vi "GetParameterValueInteger.vi"(8 "error in (no error)":errorcluster, 11 "Parameter in":refnum<class "Parameter.lvclass">) -> (0 "error out":errorcluster, 2 "Value":i32, 3 "Parameter out":refnum<class "Parameter.lvclass">)   [LabVIEW 2023, in "Easy.SequenceManagerLabVIEW.lvlib" / "Parameter.lvclass"]
uses:
  Parameter.lvclass
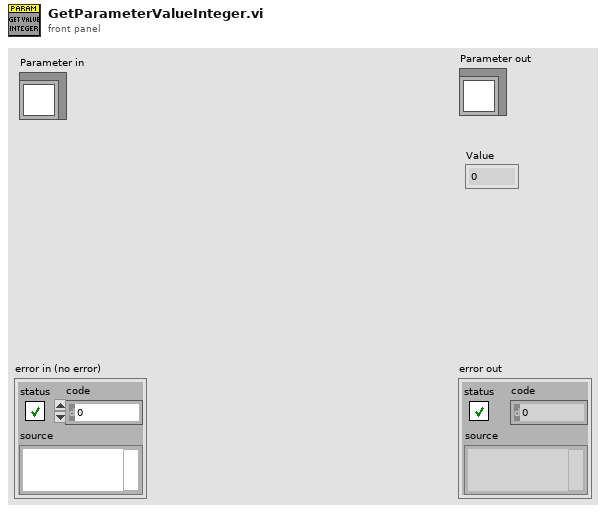
[diagram p1: front panel]
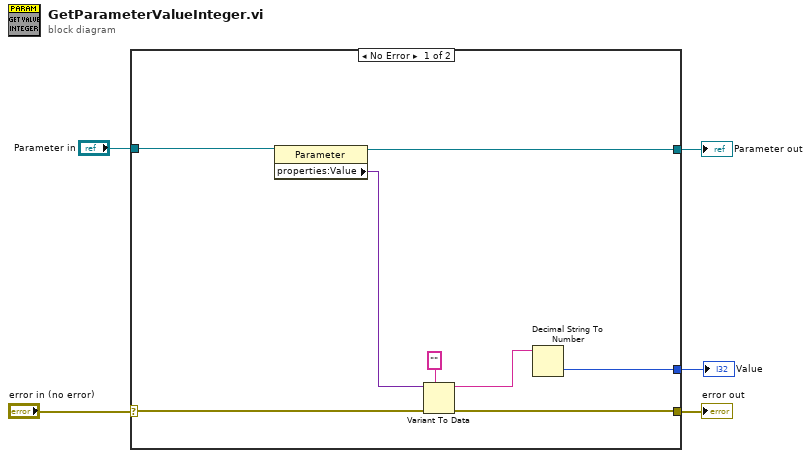
[diagram p0: block diagram]
diagram:
  n1 = case shown="No Error" "error in (no error)" {
    selector: "error in (no error)" -> [w13 w15]
    tunnel: [w10 w15] -> w4
    tunnel: "Parameter in" -> [w8 w14]
    tunnel: [w9 w14] -> w2
    tunnel: [w6 _] -> w1
    frame No Error {
      n2 = property class="Parameter"(reference=w8) -> (reference out=w9:refnum<class "Parameter.lvclass">, "properties:Value"=w11:variant)  [unwired: 1 in, 1 out]
      n3 = Variant To Data(error in=w13, type="", Variant=w11) -> (data=w7:string, error out=w10:errorcluster)
      n4 = Decimal String To Number(string=w7) -> (number=w6:i32)  [unwired: 2 in, 1 out]
    }
    frame Error {
    }
  }
  "error out" <- w4
  "Parameter out" <- w2
  "Value" <- w1
